vi "Timestamp GPIO.vi"(0 "timestamp counter value":T1, 1 "reset":bool) -> (4 "gpio timestamp fifo overflow":bool)   [LabVIEW 2023, in "GettingStarted_Common_148X_FPGA.lvlib"]
uses:
  GettingStarted_Common_148X_FPGA.lvlib
  <instrlib>/FlexRIO/CSI-2/v2/FPGA/Types/Timestamp Counter Value.ctl
  <instrlib>/_niInstr/Basic Elements/v1/FPGA/Private/Write U64 FIFO.vi
  <instrlib>/_niInstr/Basic Elements/v1/FPGA/niInstr Basic Elements v1 FPGA.lvlib
  <instrlib>/FlexRIO/CSI-2/v2/FPGA/NI CSI-2 API FPGA v2.lvlib
  <instrlib>/FlexRIO/CSI-2/v2/FPGA/subVIs/Convert GPIO Bank Timestamp to Raw Timestamp.vi
  <instrlib>/FlexRIO/CSI-2/v2/FPGA/Types/Timestamp ID.ctl
  Types/SerDes Identifier.ctl
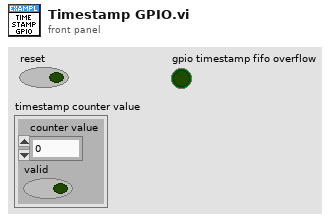
[diagram p1: front panel]
types:
  T1 = typedef "NI CSI-2 API FPGA v2.lvlib/Timestamp Counter Value.ctl" = cluster{"counter value":u64, "valid":bool}
  T2 = typedef "GettingStarted_Common_148X_FPGA.lvlib/SerDes Identifier.ctl" = enum8{"None", "SI 0 Deserializer", "SI 1 Deserializer", "SI 2 Deserializer", "SI 3 Deserializer", "SI 4 Deserializer", "SI 5 Deserializer", "SI 6 Deserializer", "SI 7 Deserializer", "SO 0 Serializer", "SO 1 Serializer", "SO 2 Serializer", "SO 3 Serializer", "SO 4 Serializer", "SO 5 Serializer", "SO 6 Serializer", "SO 7 Serializer", "SI 0 SI 1 Deserializer", "SI 2 SI 3 Deserializer", "SI 4 SI 5 Deserializer", "SI 6 SI 7 Deserializer"}
  T3 = typedef "NI CSI-2 API FPGA v2.lvlib/Timestamp ID.ctl" = enum8{"SI0 LLP", "SI1 LLP", "SI2 LLP", "SI3 LLP", "SI4 LLP", "SI5 LLP", "SI6 LLP", "SI7 LLP", "SO0 LLP", "SO1 LLP", "SO2 LLP", "SO3 LLP", "SO4 LLP", "SO5 LLP", "SO6 LLP", "SO7 LLP", "Ser0 GPIO Bank", "Ser1 GPIO Bank", "Ser2 GPIO Bank", "Ser3 GPIO Bank", "Ser4 GPIO Bank", "Ser5 GPIO Bank", "Ser6 GPIO Bank", "Ser7 GPIO Bank", "Des0 GPIO Bank", "Des1 GPIO Bank", "Des2 GPIO Bank", "Des3 GPIO Bank", "Des4 GPIO Bank", "Des5 GPIO Bank", "Des6 GPIO Bank", "Des7 GPIO Bank", "User0", "User1", "User2", "User3", "User4", "User5", "User6", "User7", "User8", "User9", "User10", "User11", "User12", "User13", "User14", "User15", "User16", "User17", "User18", "User19", "User20", "User21", "User22", "User23", "User24", "User25", "User26", "User27", "User28", "User29", "User30", "User31"}
  T4 = typedef "NI CSI-2 API FPGA v2.lvlib/GPIO Bank.ctl" = cluster{"GPIO 0":bool, "GPIO 1":bool, "GPIO 2":bool, "GPIO 3":bool, "GPIO 4":bool, "GPIO 5":bool, "GPIO 6":bool, "GPIO 7":bool, "GPIO 8":bool, "GPIO 9":bool, "GPIO 10":bool}
  T5 = typedef "NI CSI-2 API FPGA v2.lvlib/FPGA GPIO Bank Timestamp.ctl" = cluster{"valid":bool, "count":fxp<+,47,47>, "id":T3, "gpio bank":T4}
  T6 = typedef "NI CSI-2 API FPGA v2.lvlib/Raw Timestamp.ctl" = cluster{"timestamp":u64, "valid":bool}
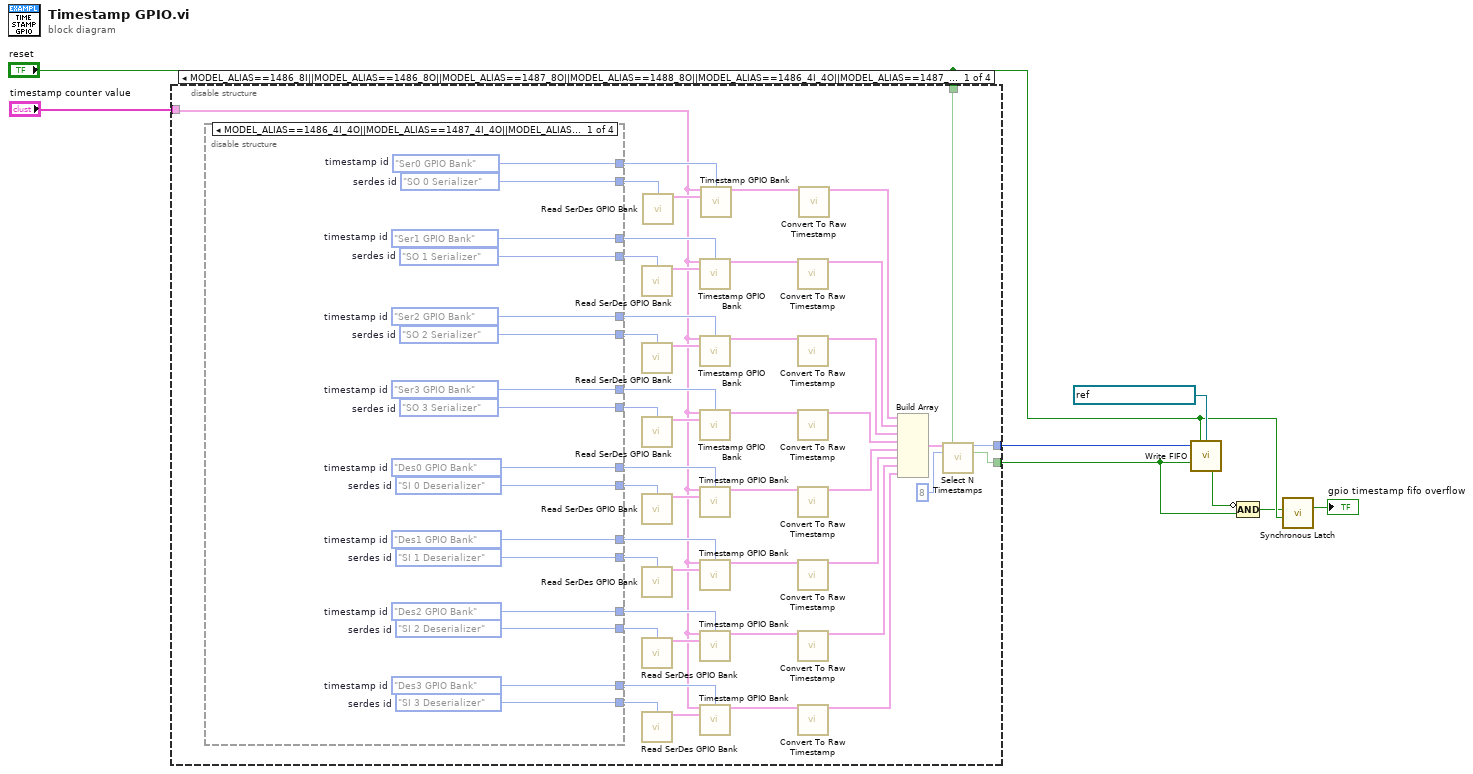
[diagram p0: block diagram]
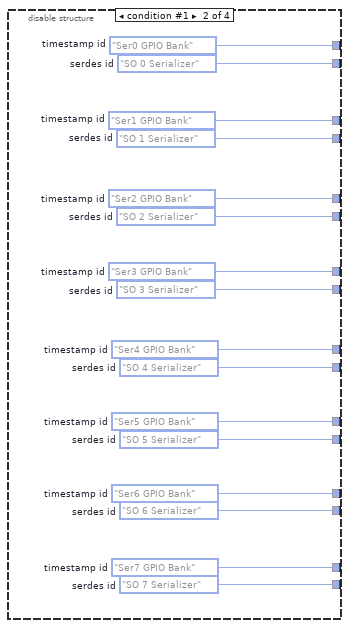
[diagram p2: hidden frame]
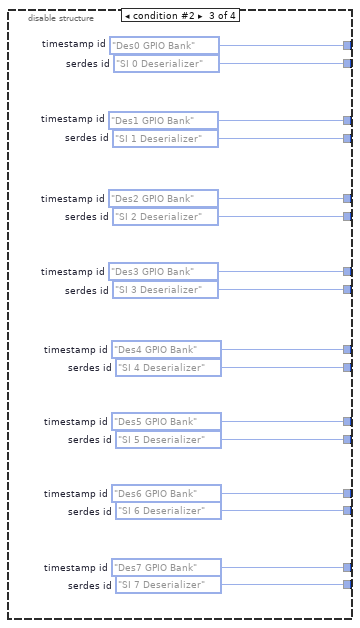
[diagram p3: hidden frame]
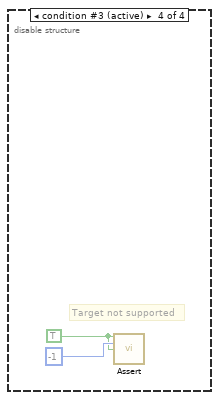
[diagram p4: hidden frame]
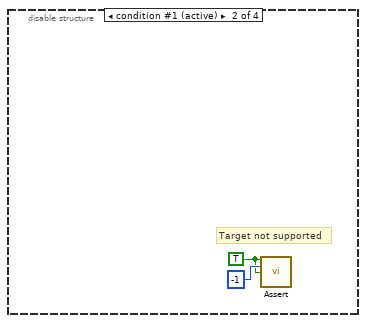
[diagram p5: hidden frame]
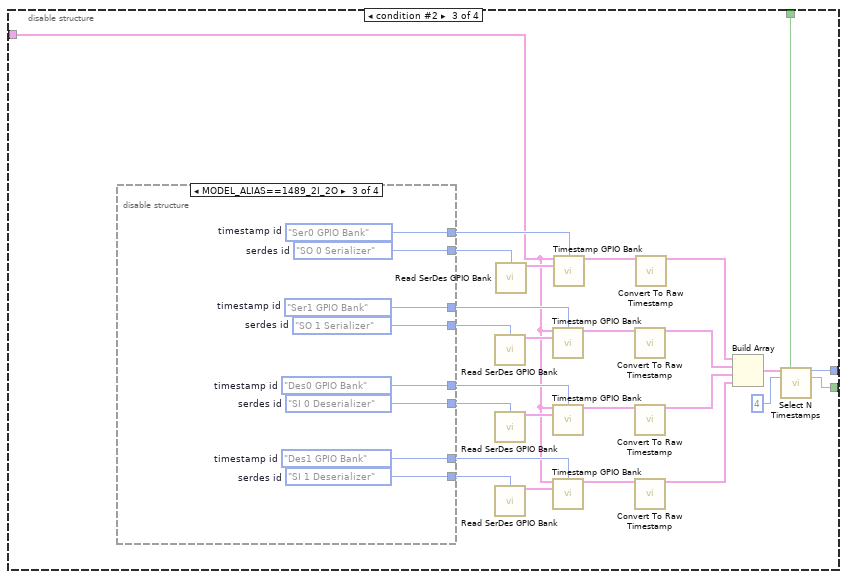
[diagram p6: hidden frame]
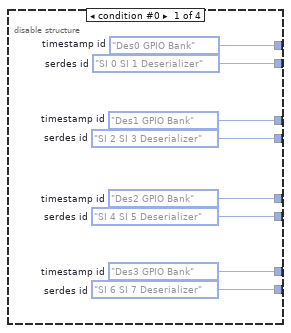
[diagram p7: hidden frame]
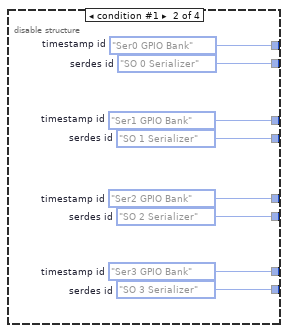
[diagram p8: hidden frame]
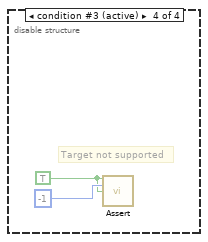
[diagram p9: hidden frame]
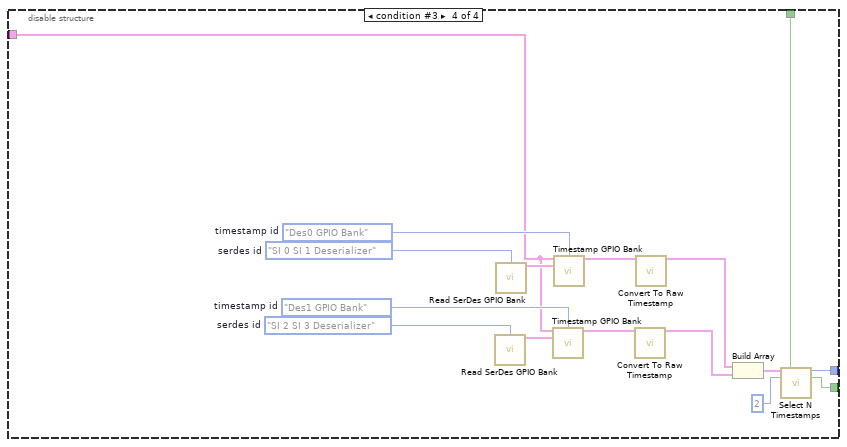
[diagram p10: hidden frame]
diagram:
  n1 = disable-structure shown="MODEL_ALIAS==1486_8I||MODEL_ALIAS==1486_8O||MODEL_ALIAS==1487_8O||MODEL_ALIAS==1488_8O||MODEL_ALIAS==1486_4I_4O||MODEL_ALIAS==1487_4I_4O||MODEL_ALIAS==1488_4I_4O" {
    disable-tunnel: "timestamp counter value" -> [w14 _ w112 w164]
    disable-tunnel: "reset" -> [w10 _ w108 w160]
    disable-tunnel: [w13 _ w111 w163] -> w3
    disable-tunnel: [w12 _ w110 w162] -> w2
    frame condition #0 {
      n2 = disable-structure shown="MODEL_ALIAS==1486_4I_4O||MODEL_ALIAS==1487_4I_4O||MODEL_ALIAS==1488_4I_4O" {
        disable-tunnel: [w70 w86 w102 _] -> w36
        disable-tunnel: [w69 w85 w101 _] -> w35
        disable-tunnel: [w68 w84 w100 _] -> w34
        disable-tunnel: [w67 w83 w99 _] -> w33
        disable-tunnel: [w66 w82 w98 _] -> w32
        disable-tunnel: [w65 w81 w97 _] -> w31
        disable-tunnel: [w64 w80 w96 _] -> w30
        disable-tunnel: [w63 w79 w95 _] -> w29
        disable-tunnel: [w62 w78 w94 _] -> w25
        disable-tunnel: [w61 w77 w93 _] -> w21
        disable-tunnel: [w60 w76 w92 _] -> w20
        disable-tunnel: [w59 w75 w91 _] -> w19
        disable-tunnel: [w58 w74 w90 _] -> w18
        disable-tunnel: [w57 w73 w89 _] -> w17
        disable-tunnel: [w56 w72 w88 _] -> w16
        disable-tunnel: [w55 w71 w87 _] -> w15
        frame condition #0 {
          w55 = SerDes_Identifier."SI 3 Deserializer"  # serdes id
          w56 = SerDes_Identifier."SI 2 Deserializer"  # serdes id
          w57 = SerDes_Identifier."SI 1 Deserializer"  # serdes id
          w58 = SerDes_Identifier."SI 0 Deserializer"  # serdes id
          w59 = SerDes_Identifier."SO 3 Serializer"  # serdes id
          w60 = SerDes_Identifier."SO 2 Serializer"  # serdes id
          w61 = SerDes_Identifier."SO 1 Serializer"  # serdes id
          w62 = SerDes_Identifier."SO 0 Serializer"  # serdes id
          w63 = Timestamp_ID."Ser0 GPIO Bank"  # timestamp id
          w64 = Timestamp_ID."Des3 GPIO Bank"  # timestamp id
          w65 = Timestamp_ID."Des2 GPIO Bank"  # timestamp id
          w66 = Timestamp_ID."Des1 GPIO Bank"  # timestamp id
          w67 = Timestamp_ID."Des0 GPIO Bank"  # timestamp id
          w68 = Timestamp_ID."Ser3 GPIO Bank"  # timestamp id
          w69 = Timestamp_ID."Ser2 GPIO Bank"  # timestamp id
          w70 = Timestamp_ID."Ser1 GPIO Bank"  # timestamp id
        }
        frame condition #1 {
          w71 = SerDes_Identifier."SO 7 Serializer"  # serdes id
          w72 = SerDes_Identifier."SO 6 Serializer"  # serdes id
          w73 = SerDes_Identifier."SO 5 Serializer"  # serdes id
          w74 = SerDes_Identifier."SO 4 Serializer"  # serdes id
          w75 = SerDes_Identifier."SO 3 Serializer"  # serdes id
          w76 = SerDes_Identifier."SO 2 Serializer"  # serdes id
          w77 = SerDes_Identifier."SO 1 Serializer"  # serdes id
          w78 = SerDes_Identifier."SO 0 Serializer"  # serdes id
          w79 = Timestamp_ID."Ser0 GPIO Bank"  # timestamp id
          w80 = Timestamp_ID."Ser7 GPIO Bank"  # timestamp id
          w81 = Timestamp_ID."Ser6 GPIO Bank"  # timestamp id
          w82 = Timestamp_ID."Ser5 GPIO Bank"  # timestamp id
          w83 = Timestamp_ID."Ser4 GPIO Bank"  # timestamp id
          w84 = Timestamp_ID."Ser3 GPIO Bank"  # timestamp id
          w85 = Timestamp_ID."Ser2 GPIO Bank"  # timestamp id
          w86 = Timestamp_ID."Ser1 GPIO Bank"  # timestamp id
        }
        frame condition #2 {
          w87 = SerDes_Identifier."SI 7 Deserializer"  # serdes id
          w88 = SerDes_Identifier."SI 6 Deserializer"  # serdes id
          w89 = SerDes_Identifier."SI 5 Deserializer"  # serdes id
          w90 = SerDes_Identifier."SI 4 Deserializer"  # serdes id
          w91 = SerDes_Identifier."SI 3 Deserializer"  # serdes id
          w92 = SerDes_Identifier."SI 2 Deserializer"  # serdes id
          w93 = SerDes_Identifier."SI 1 Deserializer"  # serdes id
          w94 = SerDes_Identifier."SI 0 Deserializer"  # serdes id
          w95 = Timestamp_ID."Des0 GPIO Bank"  # timestamp id
          w96 = Timestamp_ID."Des7 GPIO Bank"  # timestamp id
          w97 = Timestamp_ID."Des6 GPIO Bank"  # timestamp id
          w98 = Timestamp_ID."Des5 GPIO Bank"  # timestamp id
          w99 = Timestamp_ID."Des4 GPIO Bank"  # timestamp id
          w100 = Timestamp_ID."Des3 GPIO Bank"  # timestamp id
          w101 = Timestamp_ID."Des2 GPIO Bank"  # timestamp id
          w102 = Timestamp_ID."Des1 GPIO Bank"  # timestamp id
        }
        frame condition #3 (active) {
          w103 = TRUE ("assert")
          # "Target not supported"
          n3 = call <instrlib>:"Assert.vi"("assert"=w103, "error code"=-1, "enable show error"=w103) -> ()  [unwired: 13 in]
        }
      }
      n4 = call "Read SerDes GPIO Bank.vi"("serdes id"=w21) -> ("gpio bank input"=w43:T4)  [unwired: 13 in, 1 out]
      n5 = call "Read SerDes GPIO Bank.vi"("serdes id"=w20) -> ("gpio bank input"=w42:T4)  [unwired: 13 in, 1 out]
      n6 = call "Read SerDes GPIO Bank.vi"("serdes id"=w19) -> ("gpio bank input"=w41:T4)  [unwired: 13 in, 1 out]
      n7 = call "Read SerDes GPIO Bank.vi"("serdes id"=w18) -> ("gpio bank input"=w40:T4)  [unwired: 13 in, 1 out]
      n8 = call "Read SerDes GPIO Bank.vi"("serdes id"=w17) -> ("gpio bank input"=w39:T4)  [unwired: 13 in, 1 out]
      n9 = call "Read SerDes GPIO Bank.vi"("serdes id"=w16) -> ("gpio bank input"=w38:T4)  [unwired: 13 in, 1 out]
      n10 = call "Read SerDes GPIO Bank.vi"("serdes id"=w15) -> ("gpio bank input"=w37:T4)  [unwired: 13 in, 1 out]
      n11 = call "Read SerDes GPIO Bank.vi"("serdes id"=w25) -> ("gpio bank input"=w28:T4)  [unwired: 13 in, 1 out]
      n12 = call <instrlib>:"Timestamp GPIO Bank.vi"("timestamp counter value"=w14, "timestamp id"=w36, "gpio bank"=w43) -> ("gpio bank timestamp"=w54:T5)  [unwired: 12 in]
      n13 = call <instrlib>:"Timestamp GPIO Bank.vi"("timestamp counter value"=w14, "timestamp id"=w35, "gpio bank"=w42) -> ("gpio bank timestamp"=w51:T5)  [unwired: 12 in]
      n14 = call <instrlib>:"Timestamp GPIO Bank.vi"("timestamp counter value"=w14, "timestamp id"=w34, "gpio bank"=w41) -> ("gpio bank timestamp"=w50:T5)  [unwired: 12 in]
      n15 = call <instrlib>:"Timestamp GPIO Bank.vi"("timestamp counter value"=w14, "timestamp id"=w33, "gpio bank"=w40) -> ("gpio bank timestamp"=w48:T5)  [unwired: 12 in]
      n16 = call <instrlib>:"Timestamp GPIO Bank.vi"("timestamp counter value"=w14, "timestamp id"=w32, "gpio bank"=w39) -> ("gpio bank timestamp"=w47:T5)  [unwired: 12 in]
      n17 = call <instrlib>:"Timestamp GPIO Bank.vi"("timestamp counter value"=w14, "timestamp id"=w31, "gpio bank"=w38) -> ("gpio bank timestamp"=w46:T5)  [unwired: 12 in]
      n18 = call <instrlib>:"Timestamp GPIO Bank.vi"("timestamp counter value"=w14, "timestamp id"=w30, "gpio bank"=w37) -> ("gpio bank timestamp"=w45:T5)  [unwired: 12 in]
      n19 = call <instrlib>:"Timestamp GPIO Bank.vi"("timestamp counter value"=w14, "timestamp id"=w29, "gpio bank"=w28) -> ("gpio bank timestamp"=w27:T5)  [unwired: 12 in]
      n20 = call-poly <instrlib>:"Convert To Raw Timestamp.vi"("gpio bank timestamp"=w54) -> ("raw timestamp"=w53:T6)  [unwired: 14 in]
      n21 = call-poly <instrlib>:"Convert To Raw Timestamp.vi"("gpio bank timestamp"=w51) -> ("raw timestamp"=w52:T6)  [unwired: 14 in]
      n22 = call-poly <instrlib>:"Convert To Raw Timestamp.vi"("gpio bank timestamp"=w50) -> ("raw timestamp"=w49:T6)  [unwired: 14 in]
      n23 = call-poly <instrlib>:"Convert To Raw Timestamp.vi"("gpio bank timestamp"=w48) -> ("raw timestamp"=w44:T6)  [unwired: 14 in]
      n24 = call-poly <instrlib>:"Convert To Raw Timestamp.vi"("gpio bank timestamp"=w47) -> ("raw timestamp"=w24:T6)  [unwired: 14 in]
      n25 = call-poly <instrlib>:"Convert To Raw Timestamp.vi"("gpio bank timestamp"=w46) -> ("raw timestamp"=w23:T6)  [unwired: 14 in]
      n26 = call-poly <instrlib>:"Convert To Raw Timestamp.vi"("gpio bank timestamp"=w45) -> ("raw timestamp"=w22:T6)  [unwired: 14 in]
      n27 = call-poly <instrlib>:"Convert To Raw Timestamp.vi"("gpio bank timestamp"=w27) -> ("raw timestamp"=w26:T6)  [unwired: 14 in]
      n28 = Build Array(w26, w53, w52, w49, w44, w24, w23, w22) -> (w11:T6[])
      n29 = call <instrlib>:"Select N Timestamps.vi"("raw timestamps"=w11, "reset"=w10, "number of timestamps"=u8 8) -> ("timestamp"=w13:u64, "output valid"=w12:bool)  [unwired: 11 in]
    }
    frame condition #1 (active) {
      w105 = TRUE ("assert")
      # "Target not supported"
      n30 = call <instrlib>:"Assert.vi"("assert"=w105, "error code"=-1, "enable show error"=w105) -> ()  [unwired: 13 in]
    }
    frame condition #2 {
      n31 = disable-structure shown="MODEL_ALIAS==1489_2I_2O" {
        disable-tunnel: [w140 w148 w156 _] -> w123
        disable-tunnel: [w139 w147 w155 _] -> w122
        disable-tunnel: [w138 w146 w154 _] -> w121
        disable-tunnel: [w137 w145 w153 _] -> w120
        disable-tunnel: [w136 w144 w152 _] -> w116
        disable-tunnel: [w135 w143 w151 _] -> w115
        disable-tunnel: [w134 w142 w150 _] -> w114
        disable-tunnel: [w133 w141 w149 _] -> w113
        frame condition #0 {
          w133 = SerDes_Identifier."SI 6 SI 7 Deserializer"  # serdes id
          w134 = SerDes_Identifier."SI 4 SI 5 Deserializer"  # serdes id
          w135 = SerDes_Identifier."SI 2 SI 3 Deserializer"  # serdes id
          w136 = SerDes_Identifier."SI 0 SI 1 Deserializer"  # serdes id
          w137 = Timestamp_ID."Des0 GPIO Bank"  # timestamp id
          w138 = Timestamp_ID."Des3 GPIO Bank"  # timestamp id
          w139 = Timestamp_ID."Des2 GPIO Bank"  # timestamp id
          w140 = Timestamp_ID."Des1 GPIO Bank"  # timestamp id
        }
        frame condition #1 {
          w141 = SerDes_Identifier."SO 3 Serializer"  # serdes id
          w142 = SerDes_Identifier."SO 2 Serializer"  # serdes id
          w143 = SerDes_Identifier."SO 1 Serializer"  # serdes id
          w144 = SerDes_Identifier."SO 0 Serializer"  # serdes id
          w145 = Timestamp_ID."Ser0 GPIO Bank"  # timestamp id
          w146 = Timestamp_ID."Ser3 GPIO Bank"  # timestamp id
          w147 = Timestamp_ID."Ser2 GPIO Bank"  # timestamp id
          w148 = Timestamp_ID."Ser1 GPIO Bank"  # timestamp id
        }
        frame condition #2 {
          w149 = SerDes_Identifier."SI 1 Deserializer"  # serdes id
          w150 = SerDes_Identifier."SI 0 Deserializer"  # serdes id
          w151 = SerDes_Identifier."SO 1 Serializer"  # serdes id
          w152 = SerDes_Identifier."SO 0 Serializer"  # serdes id
          w153 = Timestamp_ID."Ser0 GPIO Bank"  # timestamp id
          w154 = Timestamp_ID."Des1 GPIO Bank"  # timestamp id
          w155 = Timestamp_ID."Des0 GPIO Bank"  # timestamp id
          w156 = Timestamp_ID."Ser1 GPIO Bank"  # timestamp id
        }
        frame condition #3 (active) {
          w157 = TRUE ("assert")
          # "Target not supported"
          n32 = call <instrlib>:"Assert.vi"("assert"=w157, "error code"=-1, "enable show error"=w157) -> ()  [unwired: 13 in]
        }
      }
      n33 = call "Read SerDes GPIO Bank.vi"("serdes id"=w115) -> ("gpio bank input"=w126:T4)  [unwired: 13 in, 1 out]
      n34 = call "Read SerDes GPIO Bank.vi"("serdes id"=w114) -> ("gpio bank input"=w125:T4)  [unwired: 13 in, 1 out]
      n35 = call "Read SerDes GPIO Bank.vi"("serdes id"=w113) -> ("gpio bank input"=w124:T4)  [unwired: 13 in, 1 out]
      n36 = call "Read SerDes GPIO Bank.vi"("serdes id"=w116) -> ("gpio bank input"=w119:T4)  [unwired: 13 in, 1 out]
      n37 = call <instrlib>:"Timestamp GPIO Bank.vi"("timestamp counter value"=w112, "timestamp id"=w123, "gpio bank"=w126) -> ("gpio bank timestamp"=w132:T5)  [unwired: 12 in]
      n38 = call <instrlib>:"Timestamp GPIO Bank.vi"("timestamp counter value"=w112, "timestamp id"=w122, "gpio bank"=w125) -> ("gpio bank timestamp"=w129:T5)  [unwired: 12 in]
      n39 = call <instrlib>:"Timestamp GPIO Bank.vi"("timestamp counter value"=w112, "timestamp id"=w121, "gpio bank"=w124) -> ("gpio bank timestamp"=w128:T5)  [unwired: 12 in]
      n40 = call <instrlib>:"Timestamp GPIO Bank.vi"("timestamp counter value"=w112, "timestamp id"=w120, "gpio bank"=w119) -> ("gpio bank timestamp"=w118:T5)  [unwired: 12 in]
      n41 = call-poly <instrlib>:"Convert To Raw Timestamp.vi"("gpio bank timestamp"=w132) -> ("raw timestamp"=w131:T6)  [unwired: 14 in]
      n42 = call-poly <instrlib>:"Convert To Raw Timestamp.vi"("gpio bank timestamp"=w129) -> ("raw timestamp"=w130:T6)  [unwired: 14 in]
      n43 = call-poly <instrlib>:"Convert To Raw Timestamp.vi"("gpio bank timestamp"=w128) -> ("raw timestamp"=w127:T6)  [unwired: 14 in]
      n44 = call-poly <instrlib>:"Convert To Raw Timestamp.vi"("gpio bank timestamp"=w118) -> ("raw timestamp"=w117:T6)  [unwired: 14 in]
      n45 = Build Array(w117, w131, w130, w127) -> (w109:T6[])
      n46 = call <instrlib>:"Select N Timestamps.vi"("raw timestamps"=w109, "reset"=w108, "number of timestamps"=u8 4) -> ("timestamp"=w111:u64, "output valid"=w110:bool)  [unwired: 11 in]
    }
    frame condition #3 {
      w165 = SerDes_Identifier."SI 2 SI 3 Deserializer"  # serdes id
      w166 = SerDes_Identifier."SI 0 SI 1 Deserializer"  # serdes id
      w170 = Timestamp_ID."Des0 GPIO Bank"  # timestamp id
      w171 = Timestamp_ID."Des1 GPIO Bank"  # timestamp id
      n47 = call "Read SerDes GPIO Bank.vi"("serdes id"=w165) -> ("gpio bank input"=w172:T4)  [unwired: 13 in, 1 out]
      n48 = call "Read SerDes GPIO Bank.vi"("serdes id"=w166) -> ("gpio bank input"=w169:T4)  [unwired: 13 in, 1 out]
      n49 = call <instrlib>:"Timestamp GPIO Bank.vi"("timestamp counter value"=w164, "timestamp id"=w171, "gpio bank"=w172) -> ("gpio bank timestamp"=w174:T5)  [unwired: 12 in]
      n50 = call <instrlib>:"Timestamp GPIO Bank.vi"("timestamp counter value"=w164, "timestamp id"=w170, "gpio bank"=w169) -> ("gpio bank timestamp"=w168:T5)  [unwired: 12 in]
      n51 = call-poly <instrlib>:"Convert To Raw Timestamp.vi"("gpio bank timestamp"=w174) -> ("raw timestamp"=w173:T6)  [unwired: 14 in]
      n52 = call-poly <instrlib>:"Convert To Raw Timestamp.vi"("gpio bank timestamp"=w168) -> ("raw timestamp"=w167:T6)  [unwired: 14 in]
      n53 = Build Array(w167, w173) -> (w161:T6[])
      n54 = call <instrlib>:"Select N Timestamps.vi"("raw timestamps"=w161, "reset"=w160, "number of timestamps"=u8 2) -> ("timestamp"=w163:u64, "output valid"=w162:bool)  [unwired: 11 in]
    }
  }
  n55 = call-poly <instrlib>:"Write FIFO.vi"("input data"=w3, "reset"="reset", "fifo"=refnum<k21> "GPIO Timestamps" ("FIFO In"), "input valid"=w2) -> ("ready for input"=w7:bool)  [unwired: 11 in]
  n56 = Compound Arithmetic op=AND(invert w7, w2) -> (w1:bool)
  n57 = call <instrlib>:"Synchronous Latch.vi"("clear"="reset", "set"=w1) -> ("out"=→"gpio timestamp fifo overflow":bool)  [unwired: 9 in]
